vi "Load Trigger Model GradeBinning Template.vi"(0 "VISA resource name":refnum<visa-resource-name>, 1 "Components":u32=1 min=1, 2 "Digital In Line":u32=5 min=5 max=7 step=1, 3 "Start Delay":dbl, 4 "End Delay":dbl, 5 "Upper Limit 1":dbl=1.0 min=1.0 max=4.0 step=1.0, 6 "Lower Limit 1":dbl=1.0 min=1.0 max=4.0 step=1.0, 7 "error in (no error)":errorcluster, 8 "Upper Limit 2":dbl=1.0 min=1.0 max=4.0 step=1.0, 9 "Lower Limit 2":dbl=1.0 min=1.0 max=4.0 step=1.0, 10 "Upper Limit 3":dbl=1.0 min=1.0 max=4.0 step=1.0, 11 "Lower Limit 3":dbl=1.0 min=1.0 max=4.0 step=1.0, 12 "Upper Limit 4":dbl=1.0 min=1.0 max=4.0 step=1.0, 13 "Lower Limit 4":dbl=1.0 min=1.0 max=4.0 step=1.0, 14 "Limit 1 Pattern":u32=1 min=1 max=15 step=1, 15 "Limit 2 Pattern":u32=2 min=1 max=15 step=1, 16 "Limit 3 Pattern":u32=4 min=1 max=15 step=1, 17 "Limit 4 Pattern":u32=8 min=1 max=15 step=1, 18 "Limit All Pattern":u32=15 min=1 max=15 step=1, 19 "Reading Buffer":string="defbuffer1") -> (20 "VISA resource name out":refnum<visa-resource-name>, 27 "error Out (no error)":errorcluster)   [LabVIEW 2016, in "Keithley DMM7510.lvlib"]
doc: "This VI loads a predefined trigger model configuration that sets up a grading operation."
uses:
  Keithley DMM7510.lvlib
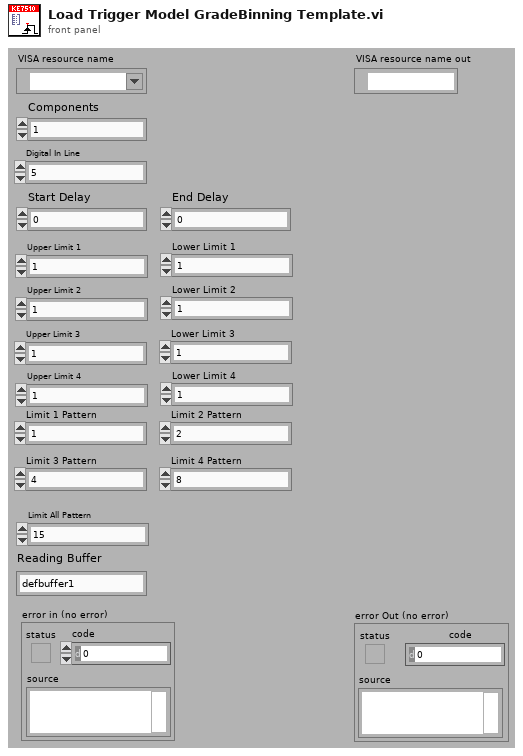
[diagram p1: front panel]
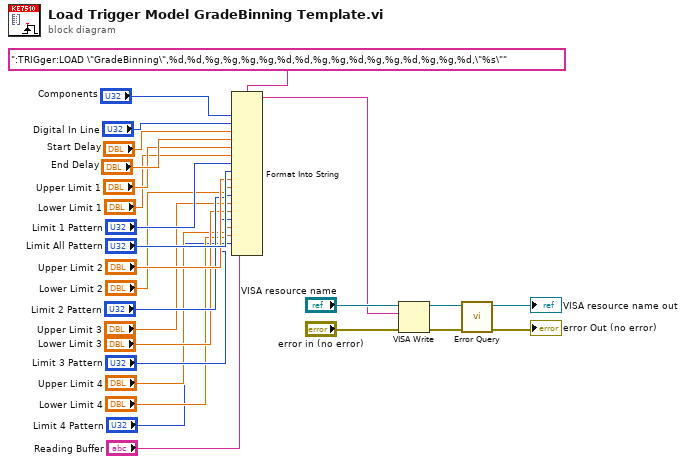
[diagram p0: block diagram]
diagram:
  n1 = Format Into String(format string=":TRIGger:LOAD \"GradeBinning\",%d,%d,%g,%g,%g,%g,%d,%d,%g,%g,%d,%g,%g,%d,%g,%g,%d,\"%s\"", "Components", "Digital In Line", "Start Delay", "End Delay", "Upper Limit 1", "Lower Limit 1", "Limit 1 Pattern", "Limit All Pattern", "Upper Limit 2", "Lower Limit 2", "Limit 2 Pattern", "Upper Limit 3", "Lower Limit 3", "Limit 3 Pattern", "Upper Limit 4", "Lower Limit 4", "Limit 4 Pattern", "Reading Buffer") -> (resulting string=w18:string)  [unwired: 2 in, 1 out]
  n2 = VISA Write(VISA resource name="VISA resource name", write buffer=w18, error in (no error)="error in (no error)") -> (VISA resource name out=w23:refnum<visa-resource-name>, error out=w19:errorcluster)  [unwired: 1 out]
  n3 = call "Error Query.vi"("error in (no error)"=w19, "VISA resource name"=w23) -> ("error out"=→"error Out (no error)":errorcluster, "VISA resource name out"=→"VISA resource name out":refnum<visa-resource-name>)  [unwired: 6 in, 2 out]
